vi "Tilt Table_student.vi"() -> ()   [LabVIEW 2012]
uses:
  <vilib>/Instr/_visa.llb/VISA Configure Serial Port (Instr).vi
  <vilib>/vision/NI_Vision_Development_Module.lvlib
panel:
  in  "View (%)":sgl=100.0 min=0 max=100
  in  "Crop Point":i32=60 min=0 max=160 step=1
  in  "Map\nColour Coding":T1={"Empty"=16448250, "Walls"=0, "Path"=3381759, "Waypoint"=16860, "Goal"=16711680}
  in  "Ball_Ranges":T2={"Hue Range"={"Lower value"=0, "Upper value"=255}, "Sat Range"={"Lower value"=0, "Upper value"=50}, "Val Range"={"Lower value"=0, "Upper value"=255}}
  in  "Wall_Ranges":T2={"Hue Range"={"Lower value"=130, "Upper value"=165}, "Sat Range"={"Lower value"=80, "Upper value"=255}, "Val Range"={"Lower value"=0, "Upper value"=255}}
  in  "Goal_Ranges":T2={"Hue Range"={"Lower value"=35, "Upper value"=55}, "Sat Range"={"Lower value"=45, "Upper value"=255}, "Val Range"={"Lower value"=0, "Upper value"=255}}
  in  "I":dbl
  in  "Controller Active":bool
  in  "Arduino Port":refnum<visa-resource-name>="COM9"
  in  "P":dbl
  out "Ball Data":T3
  in  "Allow\nDiagonals":bool
  out "Waypoints":i32[][](array[numeric])
  out "Ball Position":T4(plugin-control)
  out "Occupancy Grid":T4(plugin-control)
  out "Goal":cluster{"X Centroid":sgl, "Y Centroid":sgl} {"Y Centroid" format="%.2f"; "X Centroid" format="%.2f"}
  out "Reduced Resolution":T4(plugin-control)
  out "Frame Rate":dbl
  out "Raw Feed":T4(plugin-control)
  in  "Stop (F)":bool
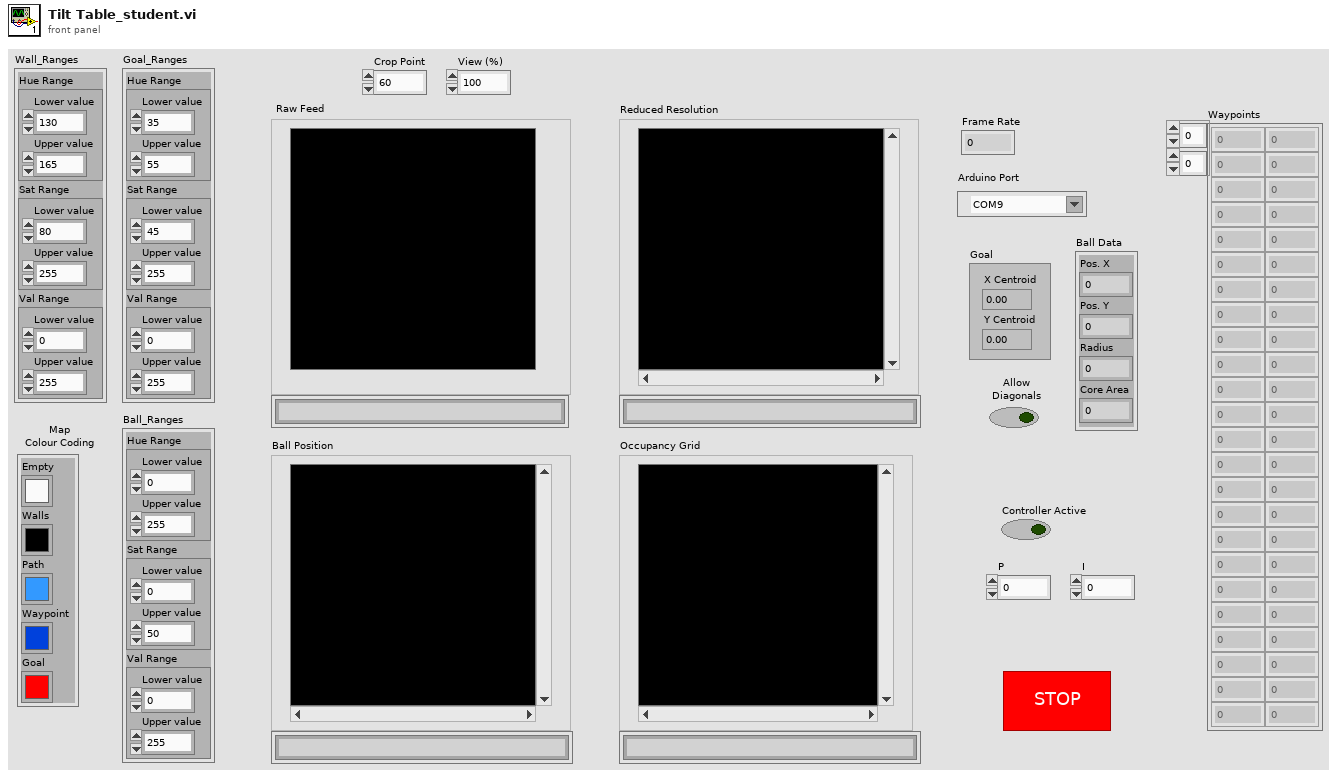
[diagram p1: front panel]
types:
  T1 = cluster{"Empty":u32, "Walls":u32, "Path":u32, "Waypoint":u32, "Goal":u32}
  T2 = cluster{"Hue Range":cluster{"Lower value":i32, "Upper value":i32}, "Sat Range":cluster{"Lower value":i32, "Upper value":i32}, "Val Range":cluster{"Lower value":i32, "Upper value":i32}}
  T3 = cluster{"Pos. X":i32, "Pos. Y":i32, "Radius":i32, "Core Area":i32}
  T4 = typedef "IMAQ Image.ctl" = refnum<image>
  T5 = typedef "Image Type" = u32
  T6 = cluster{"Pos. X":i32, "Pos. Y":i32, "Radius":i32, "Core Area":i32}[]
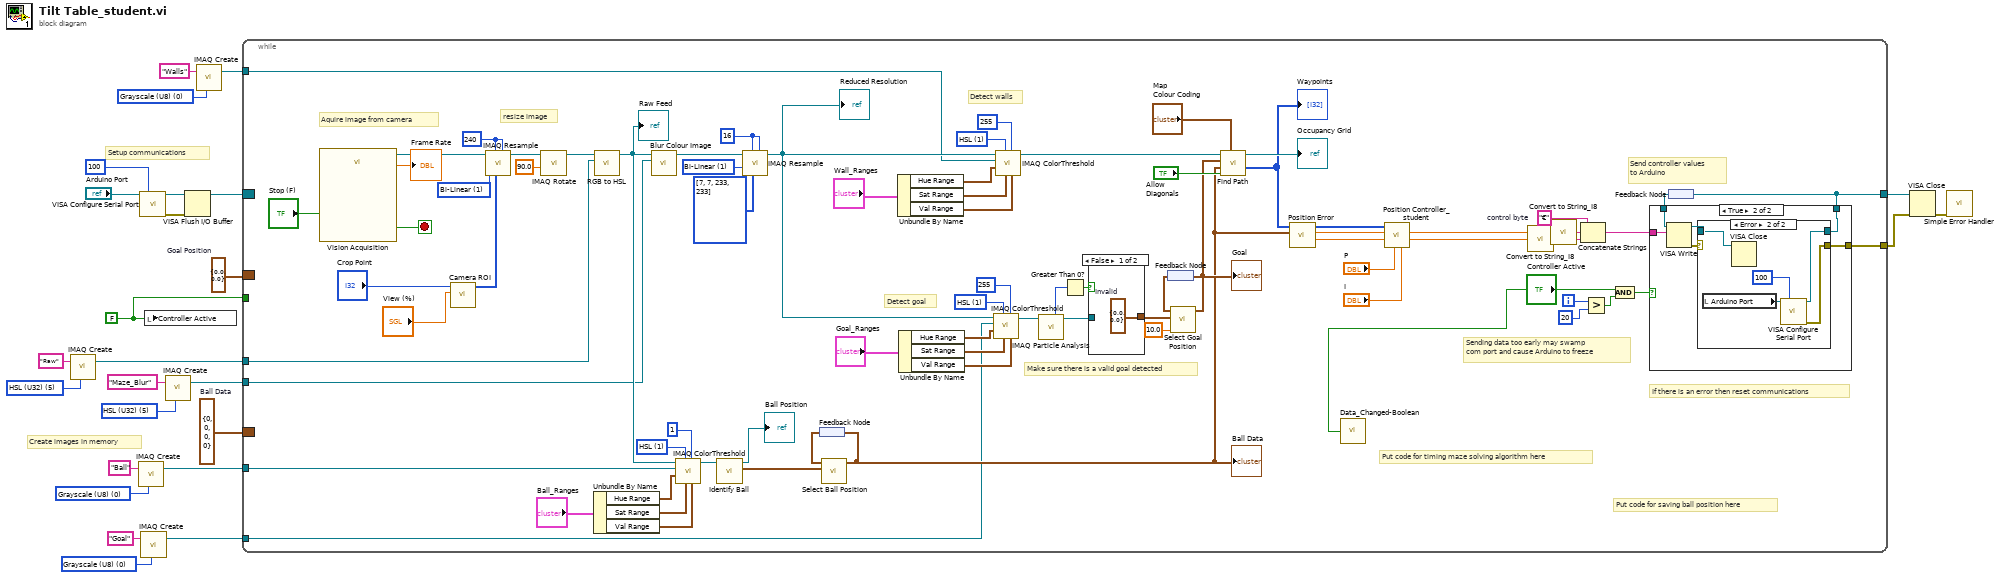
[diagram p0: block diagram]
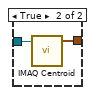
[diagram p2: hidden frame]
diagram:
  w2 = T5 0 items=["Grayscale (U8)", "Grayscale (I16)", "Grayscale (SGL)", "Complex (CSG)", "RGB (U32)", "HSL (U32)", "RGB (U64)", "Grayscale (U16)"] ("Image Type")
  w6 = T5 0 items=["Grayscale (U8)", "Grayscale (I16)", "Grayscale (SGL)", "Complex (CSG)", "RGB (U32)", "HSL (U32)", "RGB (U64)", "Grayscale (U16)"] ("Image Type")
  w10 = T5 5 items=["Grayscale (U8)", "Grayscale (I16)", "Grayscale (SGL)", "Complex (CSG)", "RGB (U32)", "HSL (U32)", "RGB (U64)", "Grayscale (U16)"] ("Image Type")
  w12 = T5 5 items=["Grayscale (U8)", "Grayscale (I16)", "Grayscale (SGL)", "Complex (CSG)", "RGB (U32)", "HSL (U32)", "RGB (U64)", "Grayscale (U16)"] ("Image Type")
  w15 = T5 0 items=["Grayscale (U8)", "Grayscale (I16)", "Grayscale (SGL)", "Complex (CSG)", "RGB (U32)", "HSL (U32)", "RGB (U64)", "Grayscale (U16)"] ("Image Type")
  w18 = FALSE ("Write")
  w25 = cluster{"X Centroid":sgl, "Y Centroid":sgl} {"X Centroid"=0.0, "Y Centroid"=0.0}  # Goal Position
  w26 = T3 {"Pos. X"=0, "Pos. Y"=0, "Radius"=0, "Core Area"=0}  # Ball Data
  # "Create images in memory"
  # "Setup communications"
  n1 = call "IMAQ Create"("Image Name"="Raw", "Image Type"=w10) -> ("New Image"=w8:T4)  [unwired: 3 in, 1 out]
  n2 = call "IMAQ Create"("Image Name"="Ball", "Image Type"=w15) -> ("New Image"=w14:T4)  [unwired: 3 in, 1 out]
  n3 = call-poly "VISA Configure Serial Port"("VISA resource name"="Arduino Port", "timeout (10sec)"=u32 100) -> ("VISA resource name out"=w22:refnum<visa-resource-name>, "error out"=w23:errorcluster)  [unwired: 7 in, 5 out]
  n4 = call "IMAQ Create"("Image Name"="Goal", "Image Type"=w6) -> ("New Image"=w4:T4)  [unwired: 3 in, 1 out]
  n5 = local write "Controller Active"(w18) -> ()
  n6 = call "IMAQ Create"("Image Name"="Maze_Blur", "Image Type"=w12) -> ("New Image"=w11:T4)  [unwired: 3 in, 1 out]
  n7 = VISA Flush I/O Buffer(VISA resource name=w22, error in (no error)=w23) -> (VISA resource name out=w21:refnum<visa-resource-name>)  [unwired: 1 in, 1 out]
  n8 = call "IMAQ Create"("Image Name"="Walls", "Image Type"=w2) -> ("New Image"=w1:T4)  [unwired: 3 in, 1 out]
  n9 = while {
    border: w26 -> [_]
    border: w25 -> [_]
    border: w21 -> [_]
    tunnel: [w45] -> w19
    tunnel: w18 -> [_]
    tunnel: [w49] -> w17
    tunnel: w14 -> [w41]
    tunnel: w11 -> [w40]
    tunnel: w8 -> [w39]
    tunnel: w4 -> [w29]
    tunnel: w1 -> [w28]
    i -> [w66]
    stop <- w103 stop-if-true
    w34 = 240 ("Y Resolution")
    w35 = u32 1 items=["Zero Order", "Bi-Linear", "Quadratic", "Cubic Spline"] ("Interpolation Type")
    w80 = "€"  # control byte
    w92 = u16 1 items=["RGB", "HSL", "HSV", "HSI"] ("Color Mode")
    w96 = u16 1 items=["RGB", "HSL", "HSV", "HSI"] ("Color Mode")
    w98 = u16 1 items=["RGB", "HSL", "HSV", "HSI"] ("Color Mode")
    w101 = 16 ("Y Resolution")
    w102 = u32 1 items=["Zero Order", "Bi-Linear", "Quadratic", "Cubic Spline"] ("Interpolation Type")
    # "Put code for saving ball position here"
    # "Put code for timing maze solving algorithm here"
    # "Detect goal"
    # "Detect walls"
    # "If there is an error then reset communications"
    # "resize image"
    # "Aquire image from camera"
    # "Make sure there is a valid goal detected"
    # "Send controller values\nto Arduino"
    # "Sending data too early may swamp\ncom port and cause Arduino to freeze"
    n10 = call "Vision Acquisition"("Stop (F)"="Stop (F)") -> ("Image Out"=w33:T4, "Frame Rate"=→"Frame Rate":dbl, "Stopped"=w103:bool)  [unwired: 23 in, 1 out]
    n11 = call "Camera ROI.vi"("View (%)"="View (%)", "Crop Point"="Crop Point") -> ("Camera ROI"=w42:i32[])  [unwired: 9 in]
    n12 = call "IMAQ Resample"("X Resolution"=w34, "Optional Rectangle"=w42, "Y Resolution"=w34, "Interpolation Type"=w35, "Image Src"=w33) -> ("Image Dst Out"=w31:T4)  [unwired: 5 in, 1 out]
    n13 = call "IMAQ Rotate"("Angle (degrees)"=sgl 90.0, "Image Src"=w31) -> ("Image Dst Out"=w32:T4)  [unwired: 8 in, 1 out]
    n14 = Unbundle By Name("Ball_Ranges") -> ("Hue Range"=w54:cluster{"Lower value":i32, "Upper value":i32}, "Sat Range"=w53:cluster{"Lower value":i32, "Upper value":i32}, "Val Range"=w52:cluster{"Lower value":i32, "Upper value":i32})
    n15 = call "RGB to HSL.vi"("Destination (HSL)"=w39, "Image (RGB)"=w32) -> ("Image Out (HSL)"=w84:T4)  [unwired: 9 in]
    "Raw Feed" <- w84
    n16 = call "Blur Colour Image.vi"("Image Dest"=w40, "Image Src"=w84) -> ("Image Dest Out"=w99:T4)  [unwired: 9 in]
    n17 = call "IMAQ ColorThreshold"("Blue or Luma or Val or Inten Range"=w52, "Replace Value"=1, "Green or Sat Range"=w53, "Color Mode"=w92, "Red or Hue Range"=w54, "Image Dst"=w41, "Image Src"=w84) -> ("Image Dst Out"=w47:T4)  [unwired: 3 in, 1 out]
    n18 = call "Identify Ball.vi"("Raw Image"=w47) -> ("Ball Data"=w88:T6, "Ball Position"=→"Ball Position":T4)  [unwired: 9 in]
    n19 = call "IMAQ Resample"("X Resolution"=w101, "Optional Rectangle"=i32[] [7, 7, 233, 233], "Y Resolution"=w101, "Interpolation Type"=w102, "Image Src"=w99) -> ("Image Dst Out"=w94:T4)  [unwired: 5 in, 1 out]
    "Reduced Resolution" <- w94
    n20 = feedback #1() -> (w89:T3)
    n21 = call "Select Ball Position.vi"("Circles Data"=w88, "Ball Data past"=w89) -> ("Ball Data out"=w81:T3)  [unwired: 9 in]
    "Ball Data" <- w81
    n22 = feedback-in #1(w81) -> ()
    n23 = Unbundle By Name("Wall_Ranges") -> ("Hue Range"=w61:cluster{"Lower value":i32, "Upper value":i32}, "Sat Range"=w60:cluster{"Lower value":i32, "Upper value":i32}, "Val Range"=w59:cluster{"Lower value":i32, "Upper value":i32})
    n24 = Unbundle By Name("Goal_Ranges") -> ("Hue Range"=w57:cluster{"Lower value":i32, "Upper value":i32}, "Sat Range"=w56:cluster{"Lower value":i32, "Upper value":i32}, "Val Range"=w55:cluster{"Lower value":i32, "Upper value":i32})
    n25 = call "IMAQ ColorThreshold"("Blue or Luma or Val or Inten Range"=w55, "Replace Value"=255, "Green or Sat Range"=w56, "Color Mode"=w96, "Red or Hue Range"=w57, "Image Dst"=w29, "Image Src"=w94) -> ("Image Dst Out"=w77:T4)  [unwired: 3 in, 1 out]
    n26 = call "IMAQ ColorThreshold"("Blue or Luma or Val or Inten Range"=w59, "Replace Value"=255, "Green or Sat Range"=w60, "Color Mode"=w98, "Red or Hue Range"=w61, "Image Dst"=w28, "Image Src"=w94) -> ("Image Dst Out"=w91:T4)  [unwired: 3 in, 1 out]
    n27 = call "IMAQ Particle Analysis"("Image"=w77) -> ("Image Out (duplicate)"=w76:T4, "Number of Particles"=w74:i32)  [unwired: 5 in, 4 out]
    n28 = Greater Than 0?(x=w74) -> (x > 0?=w75:bool)
    n29 = case shown="False" w75 {
      tunnel: [w105 w107] -> w87
      tunnel: w76 -> [_ w106]
      frame False {
        w105 = cluster{"X Centroid":sgl, "Y Centroid":sgl} {"X Centroid"=0.0, "Y Centroid"=0.0}  # Invalid
      }
      frame True {
        n30 = call "IMAQ Centroid"("Image"=w106) -> ("Centroid"=w107:cluster{"X Centroid":sgl, "Y Centroid":sgl})  [unwired: 3 in, 1 out]
      }
    }
    n31 = feedback #2() -> (w86:cluster{"X Centroid":sgl, "Y Centroid":sgl})
    n32 = call "Select Goal Position.vi"("Distance Limit (pixels)"=sgl 10.0, "Goal In"=w87, "Goal Previous"=w86) -> ("Goal Out"=w85:cluster{"X Centroid":sgl, "Y Centroid":sgl})  [unwired: 8 in]
    "Goal" <- w85
    n33 = feedback-in #2(w85) -> ()
    n34 = call "Find Path.vi"("Map Colour Coding"="Map\nColour Coding", "Diagonals"="Allow\nDiagonals", "Ball Data"=w81, "Goal"=w85, "Maze Walls"=w91) -> ("Waypoints"=w82:i32[][], "Image Out"=→"Occupancy Grid":T4)  [unwired: 4 in, 1 out]
    "Waypoints" <- w82
    n35 = call "Position Error.vi"("Ball Data in"=w81, "Waypoints"=w82) -> ("Y Error"=w71:dbl, "X Error"=w72:dbl, "Next Waypoint"=w73:i32[])  [unwired: 7 in]
    n36 = call "Data_Changed-Boolean.vi"("Data"="Controller Active") -> ()  [unwired: 1 out]
    n37 = call "Position Controller_student.vi"("I"="I", "P"="P", "Y Error"=w71, "X Error"=w72, "Next Waypoint"=w73) -> ("Controller_Outer"=w38:dbl, "Controller_Inner"=w37:dbl)  [unwired: 5 in]
    n38 = call "Convert to String_I8.vi"("Input"=w38) -> ("String (I8)"=w67:string)  [unwired: 4 in]
    n39 = call "Convert to String_I8.vi"("Input"=w37) -> ("String (I8)"=w68:string)  [unwired: 4 in]
    n40 = Concatenate Strings(w80, w68, w67) -> (w79:string)
    n41 = Greater?(x=w66, y=20) -> (0:w64:bool)
    n42 = And(x="Controller Active", y=w64) -> (x .and. y?=w63:bool)
    n43 = feedback #3() -> (w78:refnum<visa-resource-name>)
    n44 = case shown="True" w63 {
      tunnel: w79 -> [_ w114]
      tunnel: [w108 w110] -> w45
      tunnel: w78 -> [w108 w113]
      tunnel: [_ w109] -> w49
      frame False {
      }
      frame True {
        n45 = VISA Write(VISA resource name=w113, write buffer=w114) -> (VISA resource name out=w111:refnum<visa-resource-name>, error out=w112:errorcluster)  [unwired: 1 in, 1 out]
        n46 = case shown="Error" w112 {
          selector: w112 -> [w116 _]
          tunnel: w111 -> [w115 w121]
          tunnel: [w115 w119] -> w110
          tunnel: [w116 w118] -> w109
          frame No Error {
          }
          frame Error {
            n47 = local read "Arduino Port"() -> (w120:refnum<visa-resource-name>)
            n48 = VISA Close(VISA resource name=w121) -> ()  [unwired: 1 in, 1 out]
            n49 = call-poly "VISA Configure Serial Port"("VISA resource name"=w120, "timeout (10sec)"=u32 100) -> ("VISA resource name out"=w119:refnum<visa-resource-name>, "error out"=w118:errorcluster)  [unwired: 7 in, 5 out]
          }
        }
      }
    }
    n50 = feedback-in #3(w45) -> ()
  }
  n51 = VISA Close(VISA resource name=w19, error in (no error)=w17) -> (error out=w20:errorcluster)
  n52 = call <vilib>:"Simple Error Handler.vi"("error in (no error)"=w20) -> ()  [unwired: 1 in, 8 out]
